vi "Control - PID Control.vi"() -> ()   [LabVIEW 2019, in "Control Workspace Object.lvlib"]
doc: "Sample numeric display item."
uses:
  Control Workspace Object.lvlib
  <vilib>/NI VeriStand/Display Template Support/DisplayTemplateSupport.llb/cluster_Screen Item Settings.ctl
  <vilib>/NI VeriStand/Display Template Support/DisplayTemplateSupport.llb/cluster_Graph Scale Settings.ctl
  <vilib>/NI VeriStand/Display Template Support/DisplayTemplateSupport.llb/cluster_Graph Plot Settings.ctl
  NationalInstruments.VeriStand.SystemStorage
  Shared/Types/Workspace Object State Variables.ctl
  Shared/Types/UI.Refs.ctl
  Shared/Types/UDP Streaming Command Cluster.ctl
  Shared/Types/UDP Streaming State.ctl
  <vilib>/NI VeriStand/Display Template Support/DisplayTemplateSupport.llb/enum_Display Template Handler Minimal To Workspace.ctl
  Shared/Types/Workspace Object Cached Settings.ctl
  <vilib>/NI VeriStand/Execution/Workspace/WorkspaceAPI.ctl
  <vilib>/NI VeriStand/Display Template Support/DisplayTemplateSupport.llb/enum_Display Template Handler Minimal To Widget Msg.ctl
  <vilib>/NI VeriStand/Execution/Workspace/SystemStateRegEventRef.ctl
  <vilib>/NI VeriStand/Execution/Workspace/Target State Info.ctl
  <vilib>/NI VeriStand/Execution/Workspace/Target State.ctl
  <vilib>/NI VeriStand/Execution/Workspace/SystemStateEventRef.ctl
  Shared/Constants.vi
  <vilib>/NI VeriStand/Execution/Workspace/NI VeriStand - Get Multiple Channel Values.vi
  <vilib>/NI VeriStand/Execution/Workspace/NI VeriStand - Set Single Channel Value.vi
  <vilib>/NI VeriStand/Display Template Support/DisplayTemplateSupport.llb/sub_Display Template Handler Custom.vi
  Shared/Control Addon Shared.lvlib
  <vilib>/NI VeriStand/Execution/Workspace/NI_VS Workspace ExecutionAPI.lvlib
  NationalInstruments.VeriStand.ClientAPI
panel:
  in  "Manual Value":bool
  in  "Revert":bool
  in  "Apply":bool
  in  "Manual Output":dbl
  in  "Manual Control":bool
  in  "Setpoint":dbl
  in  "NIVS.System Definition Root":refnum<k24>
  in  "NIVS.Gateway IP Address":string
  in  "Hold":bool
  in  "Autoscale Y":bool=TRUE
  in  "Autoscale X":bool=TRUE
  out "Chart":waveform(dbl)[](graph)
  out "Control Name":string
  in  "Item.Data":T1
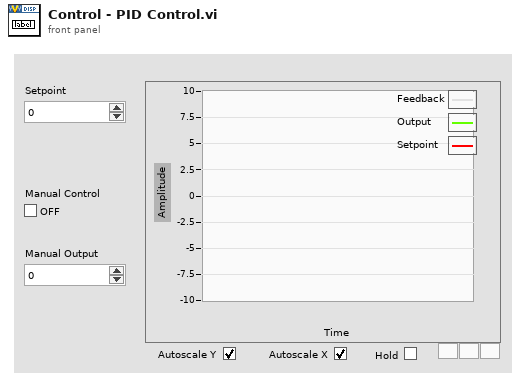
[diagram p1: front panel]
types:
  T1 = typedef "cluster_Screen Item Settings.ctl" = cluster{"Template VI":string, "Position X":i32, "Position Y":i32, "Custom":string, "Show Title Bar":bool, "ID":i32, "Always On Top":bool, "Allow Resize":bool, "Allow Minimize":bool, "Allow Close":bool, "Size to Screen":bool, "Screen.ID":i32, "State":enum16{"Normal", "New"}, "Title":string, "Window Bounds":cluster{"[0]":i16, "[1]":i16, "[2]":i16, "[3]":i16}, "Channel Ref":u64, "Unit":string, "Default Units?":bool, "Flash Limit?":bool, "Color 1":u32, "Color 2":u32, "Color 3":u32, "Color 4":u32, "Bck Color":u32, "Fore Color":u32, "Limit 1":dbl, "Limit 2":dbl, "Limit 3":dbl, "Limit 4":dbl, "Limit Mode 1":i32, "Limit Mode 2":i32, "Limit Mode 3":i32, "Limit Mode 4":i32, "Scale Precision":i32, "Scale Min":dbl, "Scale Max":dbl, "Format":i32, "Precision":i32, "Background Type":i32, "IDs":i32[], "Units":string[], "Labels":string[], "Scale Factor":dbl, "Scale Offset":dbl, "YScale Index":u32[], "XScale":T2, "YScales":T2[], "Plots":T3[], "Update Period":dbl, "History Length":dbl, "My.Ref":refnum<vi>, "Is Control?":bool, "Channel Paths":string[], "Custom Data":variant}
  T2 = typedef "cluster_Graph Scale Settings.ctl" = cluster{"Format":u8, "Precision":u8, "Fit":u8, "Label":string, "Use Default Label":bool, "Label Visible":bool, "Min":dbl, "Max":dbl}
  T3 = typedef "cluster_Graph Plot Settings.ctl" = cluster{"Bar Style":u8, "Fill To":i16, "Fill/PtColor":u32, "Line Style":u8, "Line Width":u8, "Color":u32, "Interp":u8, "Point Style":u8}
  T4 = typedef "Control Addon Shared.lvlib/Workspace Object State Variables.ctl" = cluster{"UI.Refs":T5, "Addon.GUID":string, "Addon.Name":string, "Addon.Type":enum16{"PID", "Industrial"}, "Data.UDPEngineQueue":refnum<queue>, "Data.Found?":bool, "Data.UDPChannels":string[], "Data.PreviousValues":dbl[], "Data.SlowChannels":string[], "Data.PendingChange?":bool, "CachedData.UserEvent":refnum<user-event>, "CachedData.Data":T6, "Workspace.Connected?":bool, "NIVS.SysDef":refnum<k24>, "NIVS.WorkspaceManager":T7, "NIVS.UserEventRefs":cluster{"Event Registration Refnum":refnum<event-registration>, "SystemChangeEventRef":T8}, "NIVS.SystemStateRefs":T9, "NIVS.LaunchRef":refnum<user-event>, "Setpoint Range":cluster{"Min":dbl, "Max":dbl}, "Output Range":cluster{"Min":dbl, "Max":dbl}}
  T5 = typedef "Control Addon Shared.lvlib/UI.Refs.ctl" = cluster{"Chart":refnum<vi>, "Manual Value":refnum<vi>, "Manual Output":refnum<vi>, "Revert":refnum<vi>, "Apply":refnum<vi>, "Setpoint":refnum<vi>, "Autoscale X":refnum<vi>, "Autoscale Y":refnum<vi>, "Hold":refnum<vi>, "Manual Control":refnum<vi>}
  T6 = typedef "Control Addon Shared.lvlib/Workspace Object Cached Settings.ctl" = cluster{"Path":string}
  T7 = typedef "NI_VS Workspace ExecutionAPI.lvlib/WorkspaceAPI.ctl" = refnum<k24>
  T8 = typedef "NI_VS Workspace ExecutionAPI.lvlib/SystemStateRegEventRef.ctl" = refnum<event-registration>
  T9 = typedef "NI_VS Workspace ExecutionAPI.lvlib/SystemStateEventRef.ctl" = cluster{"CustDatRef":refnum<user-event>, "EvtRef":refnum<k27>, "Target State User Event":refnum<user-event>}
  T10 = typedef "enum_Display Template Handler Minimal To Workspace.ctl" = cluster{"Operation":enum16{"SetCustomData", "DeleteItem"}, "Data":variant}
  T11 = typedef "enum_Display Template Handler Minimal To Widget Msg.ctl" = enum16{"Stop", "LaunchConfigDialog"}
  T12 = typedef "Control Addon Shared.lvlib/UDP Streaming Command Cluster.ctl" = cluster{"Action":T13, "Channels":string[]}
  T13 = typedef "Control Addon Shared.lvlib/UDP Streaming State.ctl" = enum8{"Idle", "Start Acq", "Run", "Stop Acq", "Exit"}
  T14 = cluster{"Event Registration Refnum":refnum<event-registration>, "SystemChangeEventRef":T8}
  T15 = typedef "NI_VS Workspace ExecutionAPI.lvlib/SystemState.ctl" = u8
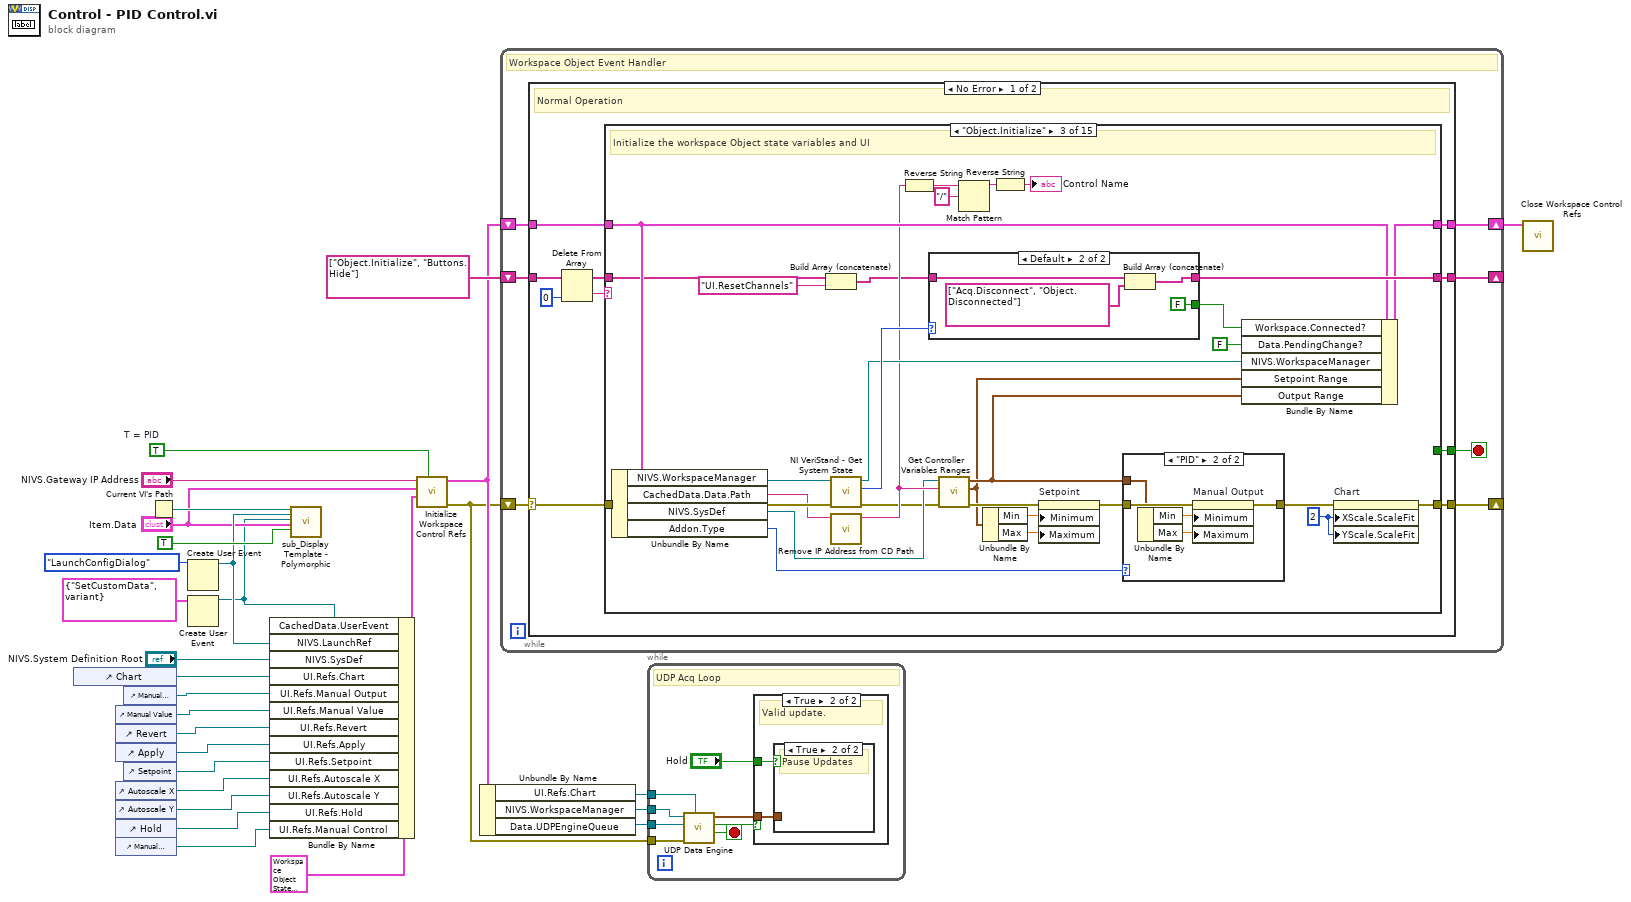
[diagram p0: block diagram]
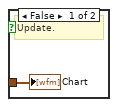
[diagram p3: hidden frame]
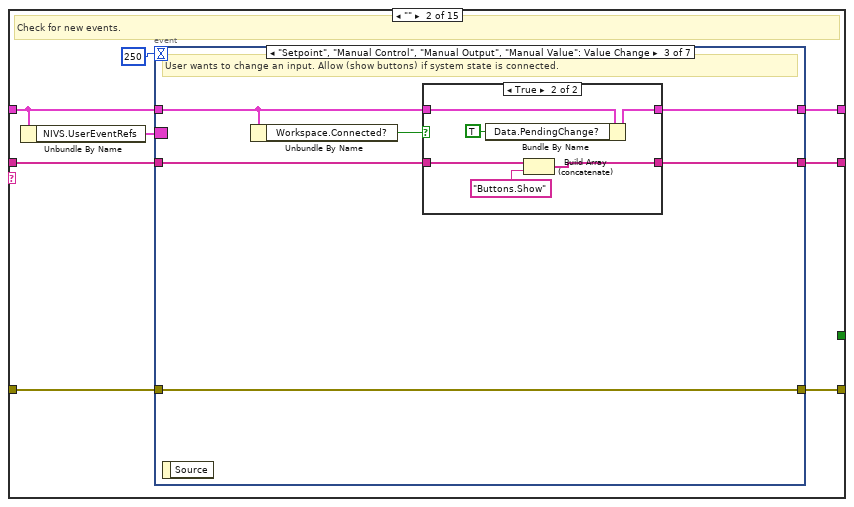
[diagram p5: hidden frame]
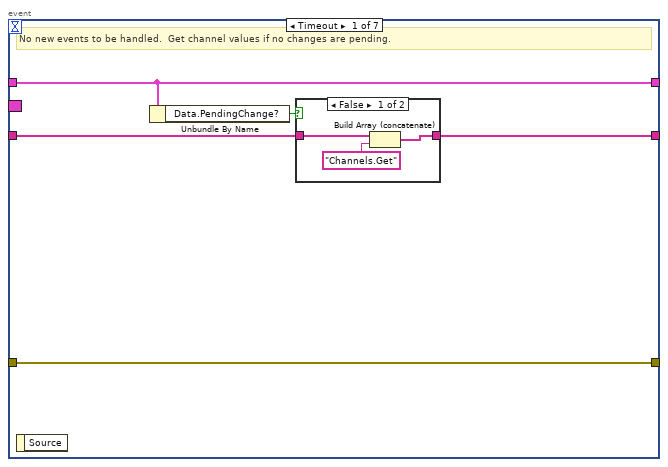
[diagram p6: hidden frame]
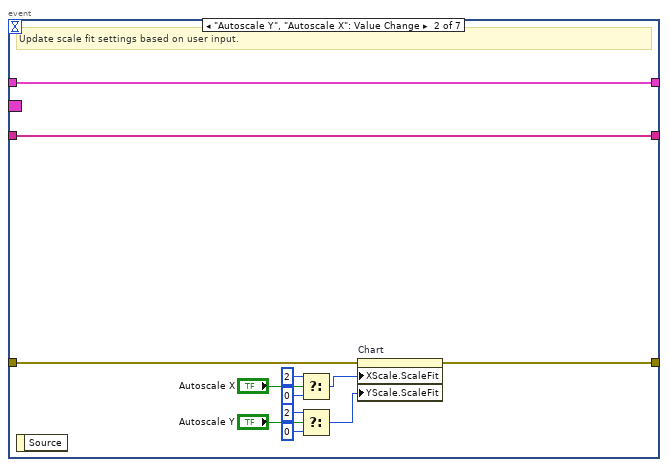
[diagram p8: hidden frame]
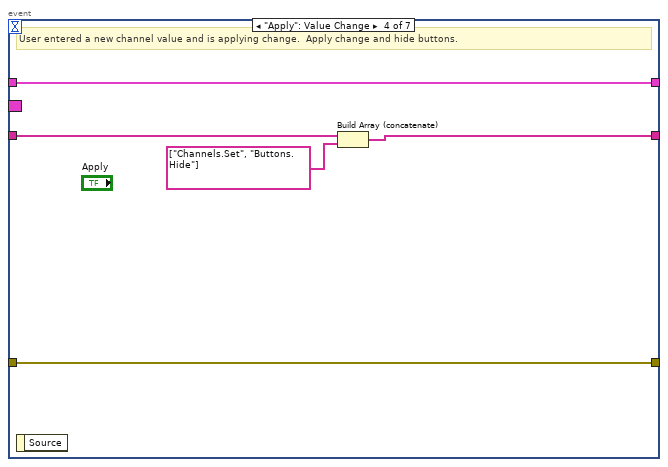
[diagram p10: hidden frame]
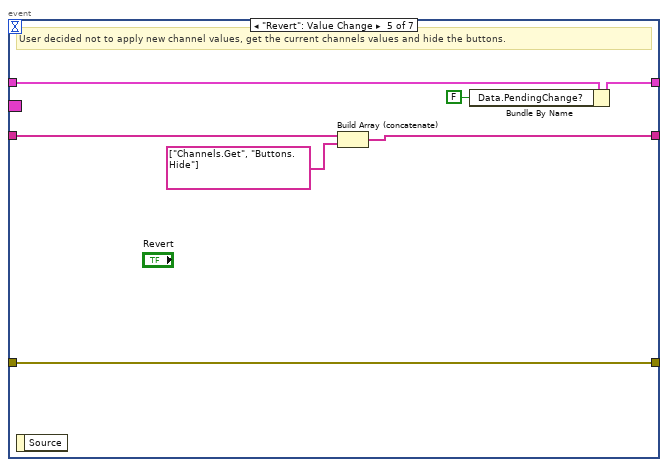
[diagram p11: hidden frame]
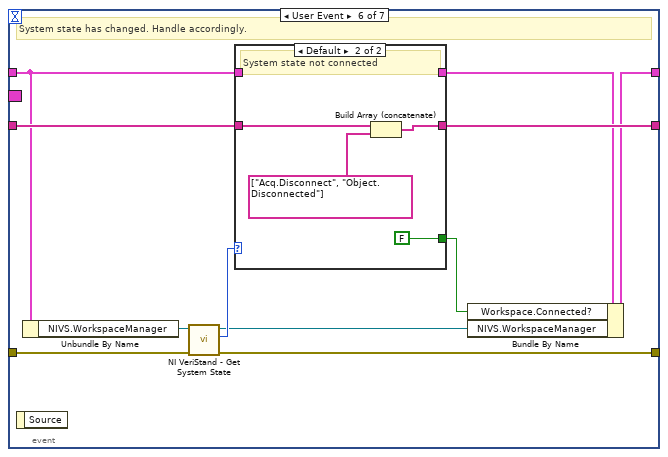
[diagram p12: hidden frame]
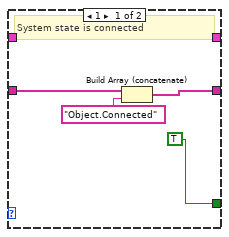
[diagram p13: hidden frame]
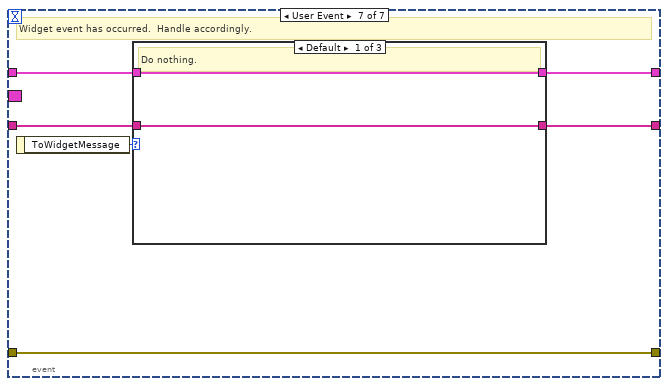
[diagram p14: hidden frame]
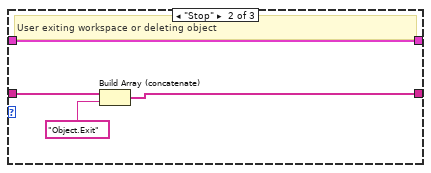
[diagram p15: hidden frame]
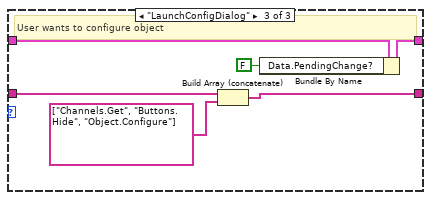
[diagram p16: hidden frame]
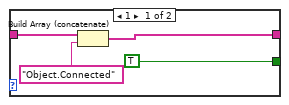
[diagram p18: hidden frame]
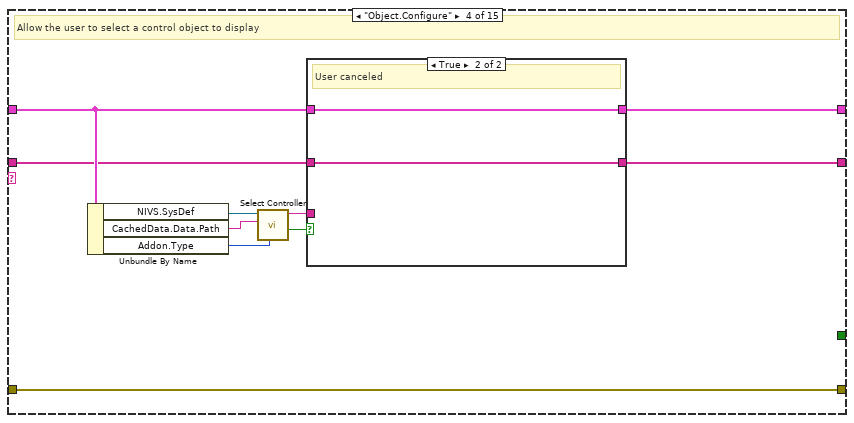
[diagram p19: hidden frame]
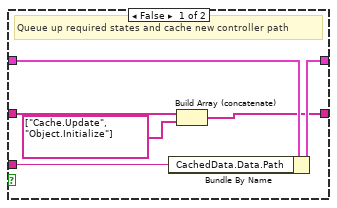
[diagram p20: hidden frame]
diagram:
  w11 = TRUE  # T = PID
  n1 = control-ref of="Chart"() -> (w17:refnum<vi>)
  n2 = control-ref of="Manual Value"() -> (w15:refnum<vi>)
  n3 = control-ref of="Revert"() -> (w14:refnum<vi>)
  n4 = control-ref of="Apply"() -> (w13:refnum<vi>)
  n5 = control-ref of="Autoscale X"() -> (w2:refnum<vi>)
  n6 = control-ref of="Autoscale Y"() -> (w3:refnum<vi>)
  n7 = control-ref of="Hold"() -> (w4:refnum<vi>)
  n8 = control-ref of="Manual Control"() -> (w1:refnum<vi>)
  n9 = control-ref of="Manual Output"() -> (w16:refnum<vi>)
  n10 = control-ref of="Setpoint"() -> (w5:refnum<vi>)
  n11 = Current VI's Path() -> (path=w27:path)
  n12 = Create User Event(user event datatype=enum_Display_Template_Handler_Minimal_To_Widget_Msg."LaunchConfigDialog" ("ToWidgetMessage")) -> (user event=w12:refnum<user-event>)  [unwired: 1 in, 1 out]
  n13 = Create User Event(user event datatype=T10 {"Operation"=enum."SetCustomData", "Data"=variant} ("Data")) -> (user event=w7:refnum<user-event>)  [unwired: 1 in, 1 out]
  n14 = Bundle By Name(cluster=T4 {"UI.Refs"={"Chart"=refnum, "Manual Value"=refnum, "Manual Output"=refnum, "Revert"=refnum, "Apply"=refnum, "Setpoint"=refnum, "Autoscale X"=refnum, "Autoscale Y"=refnum, "Hold"=refnum, "Manual Control"=refnum}, "Addon.GUID"="", "Addon.Name"="", "Addon.Type"=enum."PID", "Data.UDPEngineQueue"=refnum, "Data.Found?"=FALSE, "Data.UDPChannels"=[], "Data.PreviousValues"=[], "Data.SlowChannels"=[], "Data.PendingChange?"=FALSE, "CachedData.UserEvent"=refnum, "CachedData.Data"={"Path"=""}, "Workspace.Connected?"=FALSE, "NIVS.SysDef"=refnum, "NIVS.WorkspaceManager"=refnum, "NIVS.UserEventRefs"={"Event Registration Refnum"=refnum, "SystemChangeEventRef"=refnum}, "NIVS.SystemStateRefs"={"CustDatRef"=refnum, "EvtRef"=refnum, "Target State User Event"=refnum}, "NIVS.LaunchRef"=refnum, "Setpoint Range"={"Min"=0.0, "Max"=0.0}, "Output Range"={"Min"=0.0, "Max"=0.0}}, "CachedData.UserEvent"=w7, "NIVS.LaunchRef"=w12, "NIVS.SysDef"="NIVS.System Definition Root", "UI.Refs.Chart"=w17, "UI.Refs.Manual Output"=w16, "UI.Refs.Manual Value"=w15, "UI.Refs.Revert"=w14, "UI.Refs.Apply"=w13, "UI.Refs.Setpoint"=w5, "UI.Refs.Autoscale X"=w2, "UI.Refs.Autoscale Y"=w3, "UI.Refs.Hold"=w4, "UI.Refs.Manual Control"=w1) -> (w9:T4)
  n15 = call-poly <vilib>:"sub_Display Template - Polymorphic.vi"("Parent.Path"=w27, "ToWidgetEvent"=w12, "ToWorkspace"=w7, "Item.Data"="Item.Data", "Resizable"=TRUE) -> ()  [unwired: 1 in, 14 out]
  n16 = call "Initialize Workspace Control Refs.vi"("T = PID"=w11, "State Variables in"=w9, "Item.Data"="Item.Data", "NIVS.Gateway IP Address"="NIVS.Gateway IP Address") -> ("error out"=w6:errorcluster, "State Variables out"=w20:T4)  [unwired: 6 in]
  n17 = Unbundle By Name(w20) -> ("UI.Refs.Chart"=w22:refnum<vi>, "NIVS.WorkspaceManager"=w21:T7, "Data.UDPEngineQueue"=w19:refnum<queue>)
  n18 = while {
    shift-right: [w34] -> _
    shift-left: string[] ["Object.Initialize", "Buttons.Hide"] -> [w35]
    shift-right: [w32] -> w24
    shift-left: w20 -> [w31]
    shift-right: [w33] -> _
    shift-left: w6 -> [w30]
    stop <- w36 stop-if-true
    # "Workspace Object Event Handler"
    n19 = case shown="No Error" w30 {
      selector: w30 -> [w37 w406]
      tunnel: [w46 _] -> w36
      tunnel: w35 -> [w44 w414]
      tunnel: [w41 w414] -> w34
      tunnel: [w40 w411] -> w33
      tunnel: [w39 w413] -> w32
      tunnel: w31 -> [w38 w413]
      frame No Error {
        # "Normal Operation"
        n20 = Delete From Array(array=w44, index=0) -> (deleted portion=w43:string, array with subset deleted=w42:string[])  [unwired: 1 in]
        n21 = case shown="\"Object.Initialize\"" w43 {
          tunnel: [_ _ _ _ _ _ TRUE _ _ _ _ _ _ _ _] -> w46
          tunnel: [w49 w56 w171 w191 w219 w245 w255 w262 w270 w272 w284 w290 w305 w365 w404] -> w41
          tunnel: w37 -> [w48 w54 w172 w197 w212 w240 w250 w261 w265 w277 w280 w286 w302 w353 w403]
          tunnel: w42 -> [w49 w55 w145 w190 w228 w245 w255 w262 w270 w278 w284 w290 w305 w365 w404]
          tunnel: w38 -> [w47 w50 w162 w195 w227 w242 w247 w258 w269 w274 w283 w289 w295 w351 w402]
          tunnel: [w48 w53 w157 w197 w207 w241 w249 w261 w264 w276 w279 w285 w301 w352 w403] -> w40
          tunnel: [w47 w52 w166 w194 w209 w243 w247 w258 w269 w274 w283 w289 w300 w350 w402] -> w39
          frame Default {
            # "Do nothing."
          }
          frame "" {
            # "Check for new events."
            n22 = Unbundle By Name(w50) -> ("NIVS.UserEventRefs"=w51:T14)
            n23 = event shown="[2] \"Setpoint\", \"Manual Control\", \"Manual Output\", \"Manual Value\": Value Change" {
              selector: w51 -> [_ _ _ _ _ _ _]
              dyn-events: _ -> [_ _ _ _ _ _ _]
              timeout: 250 -> [_ _ _ _ _ _ _]
              tunnel: [w60 w78 w81 w93 w101 w111 w130] -> w56
              tunnel: w55 -> [w61 w78 w82 w94 w102 w112 w129]
              tunnel: w54 -> [w62 w72 w84 w97 w104 w115 w128]
              tunnel: [w62 w71 w84 w97 w104 w114 w128] -> w53
              tunnel: [w59 w77 w83 w96 w99 w110 w126] -> w52
              tunnel: w50 -> [w59 w77 w80 w96 w100 w107 w127]
              event Timeout {
                # "No new events to be handled.  Get channel values if no changes are pending."
                n24 = event-data() -> ()  [unwired: 2 out]
                n25 = Unbundle By Name(w59) -> ("Data.PendingChange?"=w58:bool)
                n26 = case shown="False" w58 {
                  tunnel: w61 -> [w64 w66]
                  tunnel: [w63 w66] -> w60
                  frame False {
                    n27 = Build Array (concatenate)(w64, "Channels.Get") -> (w63:string[])
                  }
                  frame True {
                  }
                }
              }
              event "Autoscale Y", "Autoscale X": Value Change {
                # "Update scale fit settings based on user input."
                n28 = event-data() -> ()  [unwired: 2 out]
                n29 = Select(t=u8 2, s="Autoscale X", f=u8 0 ("X Scale.Scale Fit")) -> (s? t:f=w74:u8)
                n30 = Select(t=u8 2, s="Autoscale Y", f=u8 0 ("X Scale.Scale Fit")) -> (s? t:f=w67:u8)
                n31 = property on="Chart" class="WFChart (strict)"(error in=w72, "XScale.ScaleFit"=w74, "YScale.ScaleFit"=w67) -> (error out=w71:errorcluster)  [unwired: 1 in, 1 out]
              }
              event "Setpoint", "Manual Control", "Manual Output", "Manual Value": Value Change {
                # "User wants to change an input. Allow (show buttons) if system state is connected."
                n32 = event-data() -> ()  [unwired: 2 out]
                n33 = Unbundle By Name(w80) -> ("Workspace.Connected?"=w79:bool)
                n34 = case shown="True" w79 {
                  tunnel: w80 -> [w85 w91]
                  tunnel: [w85 w90] -> w83
                  tunnel: w82 -> [w86 w89]
                  tunnel: [w86 w87] -> w81
                  frame False {
                  }
                  frame True {
                    n35 = Bundle By Name(cluster=w91, "Data.PendingChange?"=TRUE ("Pending Change?")) -> (w90:T4)
                    n36 = Build Array (concatenate)(w89, "Buttons.Show") -> (w87:string[])
                  }
                }
              }
              event "Apply": Value Change {
                # "User entered a new channel value and is applying change.  Apply change and hide buttons."
                n37 = event-data() -> ()  [unwired: 2 out]
                n38 = Build Array (concatenate)(w94, string[] ["Channels.Set", "Buttons.Hide"]) -> (w93:string[])
              }
              event "Revert": Value Change {
                # "User decided not to apply new channel values, get the current channels values and hide the buttons."
                n39 = event-data() -> ()  [unwired: 2 out]
                n40 = Build Array (concatenate)(w102, string[] ["Channels.Get", "Buttons.Hide"]) -> (w101:string[])
                n41 = Bundle By Name(cluster=w100, "Data.PendingChange?"=FALSE ("Pending Change?")) -> (w99:T4)
              }
              event User Event {
                # "System state has changed. Handle accordingly."
                n42 = event-data() -> ()  [unwired: 2 out]
                n43 = Unbundle By Name(w107) -> ("NIVS.WorkspaceManager"=w106:T7)
                n44 = call <vilib>:"NI VeriStand - Get System State.vi"("error in (no error)"=w115, "WorkspaceManager in"=w106) -> ("error out"=w114:errorcluster, "System State"=w113:T15, "WorkspaceManager  out"=w105:T7)  [unwired: 5 in, 2 out]
                n45 = case shown="Default" w113 {
                  tunnel: w112 -> [w120 w125]
                  tunnel: [w119 w124] -> w111
                  tunnel: [w117 w123] -> w109
                  tunnel: w107 -> [w117 w123]
                  tunnel: [TRUE FALSE] -> w108
                  frame 1 {
                    # "System state is connected"
                    n46 = Build Array (concatenate)(w120, "Object.Connected") -> (w119:string[])
                  }
                  frame Default {
                    # "System state not connected"
                    n47 = Build Array (concatenate)(w125, string[] ["Acq.Disconnect", "Object.Disconnected"]) -> (w124:string[])
                  }
                }
                n48 = Bundle By Name(cluster=w109, "Workspace.Connected?"=w108, "NIVS.WorkspaceManager"=w105) -> (w110:T4)
              }
              event User Event {
                # "Widget event has occurred.  Handle accordingly."
                n49 = event-data() -> ("ToWidgetMessage"=w131:T11)  [unwired: 1 out]
                n50 = case shown="Default" w131 {
                  tunnel: [w133 w136 w142] -> w130
                  tunnel: w129 -> [w133 w137 w143]
                  tunnel: w127 -> [w132 w134 w139]
                  tunnel: [w132 w134 w138] -> w126
                  frame Default {
                    # "Do nothing."
                  }
                  frame "Stop" {
                    # "User exiting workspace or deleting object"
                    n51 = Build Array (concatenate)(w137, "Object.Exit") -> (w136:string[])
                  }
                  frame "LaunchConfigDialog" {
                    # "User wants to configure object"
                    n52 = Build Array (concatenate)(w143, string[] ["Channels.Get", "Buttons.Hide", "Object.Configure"]) -> (w142:string[])
                    n53 = Bundle By Name(cluster=w139, "Data.PendingChange?"=FALSE ("Pending Change?")) -> (w138:T4)
                  }
                }
              }
            }
          }
          frame "Object.Initialize" {
            w164 = u8 2 ("X Scale.Scale Fit")
            # "Initialize the workspace Object state variables and UI"
            n54 = Unbundle By Name(w162) -> ("NIVS.WorkspaceManager"=w161:T7, "CachedData.Data.Path"=w155:string, "NIVS.SysDef"=w158:refnum<k24>, "Addon.Type"=w149:enum16{"PID", "Industrial"})
            n55 = Build Array (concatenate)(w145, "UI.ResetChannels") -> (w144:string[])
            n56 = call <vilib>:"NI VeriStand - Get System State.vi"("error in (no error)"=w172, "WorkspaceManager in"=w161) -> ("error out"=w156:errorcluster, "System State"=w173:T15, "WorkspaceManager  out"=w160:T7)  [unwired: 5 in, 2 out]
            n57 = call "Remove IP Address from CD Path.vi"("CD Path"=w155) -> ("Path"=w159:string)  [unwired: 10 in]
            n58 = Reverse String(1:w159) -> (0:w170:string)
            n59 = case shown="Default" w173 {
              tunnel: w144 -> [w183 w187]
              tunnel: [w182 w186] -> w171
              tunnel: [TRUE FALSE] -> w165
              frame 1 {
                n60 = Build Array (concatenate)(w183, "Object.Connected") -> (w182:string[])
              }
              frame Default {
                n61 = Build Array (concatenate)(w187, string[] ["Acq.Disconnect", "Object.Disconnected"]) -> (w186:string[])
              }
            }
            n62 = call "Get Controller Variables Ranges.vi"("error in (no error)"=w156, "Path"=w159, "NIVS.SysDef Ref"=w158) -> ("error out"=w154:errorcluster, "Setpoint Range"=w147:cluster{"Min":dbl, "Max":dbl}, "Output Range"=w148:cluster{"Min":dbl, "Max":dbl})  [unwired: 6 in]
            n63 = Match Pattern(string=w170, regular expression="/") -> (before substring=w167:string)  [unwired: 1 in, 3 out]
            n64 = Unbundle By Name(w147) -> ("Min"=w153:dbl, "Max"=w152:dbl)
            n65 = Reverse String(1:w167) -> (0:→"Control Name":string)
            n66 = property on="Setpoint" class="DigNum (strict)"(error in=w154, "Minimum"=w153, "Maximum"=w152) -> (error out=w151:errorcluster)  [unwired: 1 in, 1 out]
            n67 = case shown="\"PID\"" w149 {
              tunnel: w151 -> [w174 w179]
              tunnel: [w174 w178] -> w150
              tunnel: w148 -> [_ w177]
              frame Default {
              }
              frame "PID" {
                n68 = Unbundle By Name(w177) -> ("Min"=w176:dbl, "Max"=w175:dbl)
                n69 = property on="Manual Output" class="DigNum (strict)"(error in=w179, "Minimum"=w176, "Maximum"=w175) -> (error out=w178:errorcluster)  [unwired: 1 in, 1 out]
              }
            }
            n70 = Bundle By Name(cluster=w162, "Workspace.Connected?"=w165, "Data.PendingChange?"=FALSE ("Pending Change?"), "NIVS.WorkspaceManager"=w160, "Setpoint Range"=w147, "Output Range"=w148) -> (w166:T4)
            n71 = property on="Chart" class="WFChart (strict)"(error in=w150, "XScale.ScaleFit"=w164, "YScale.ScaleFit"=w164) -> (error out=w157:errorcluster)  [unwired: 1 in, 1 out]
          }
          frame "Object.Configure" {
            # "Allow the user to select a control object to display"
            n72 = Unbundle By Name(w195) -> ("NIVS.SysDef"=w189:refnum<k24>, "CachedData.Data.Path"=w196:string, "Addon.Type"=w188:enum16{"PID", "Industrial"})
            n73 = call "Select Controller.vi"("Type"=w188, "CD Path"=w196, "NIVS.System Definition Root"=w189) -> ("Cancelled?"=w193:bool, "Custom Device Path Out"=w192:string)  [unwired: 6 in, 1 out]
            n74 = case shown="True" w193 {
              tunnel: w195 -> [w203 w204]
              tunnel: [w202 w204] -> w194
              tunnel: w192 -> [w201 _]
              tunnel: [w199 w205] -> w191
              tunnel: w190 -> [w200 w205]
              frame False {
                # "Queue up required states and cache new controller path"
                n75 = Bundle By Name(cluster=w203, "CachedData.Data.Path"=w201) -> (w202:T4)
                n76 = Build Array (concatenate)(w200, string[] ["Cache.Update", "Object.Initialize"]) -> (w199:string[])
              }
              frame True {
                # "User canceled"
              }
            }
          }
          frame "Object.Connected" {
            w216 = "/" ("string")
            # "System state is Connected. Get path to required channels and start UDP acquisition if channels found."
            n77 = Unbundle By Name(w227) -> ("NIVS.SysDef"=w213:refnum<k24>, "CachedData.Data.Path"=w226:string, "Addon.Name"=w214:string, "Addon.GUID"=w211:string)
            n78 = global read "Constants.vi" "Name.ManualControl"() -> (w225:string)
            n79 = global read "Constants.vi" "Name.Channels"() -> (w215:string)
            n80 = call "Remove IP Address from CD Path.vi"("CD Path"=w226) -> ("Path"=w224:string)  [unwired: 10 in]
            n81 = Concatenate Strings(w224, w216, w215, w216, w225) -> (w223:string)
            n82 = Concatenate Strings(w224, w216, w215, w216, w214) -> (w222:string)
            n83 = call "Get Dependent Nodes from SysDef Root.vi"("error in (no error)"=w212, "GUID"=w211, "Path"=w224, "SysDef Ref"=w213) -> ("error out"=w208:errorcluster, "Channels"=w218:string[], "Found"=w206:bool)  [unwired: 5 in]
            n84 = Index Array(array=w218, index=2) -> (element=w220:string)
            n85 = Build Array(w220, w223, w222) -> (w217:string[])
            n86 = Bundle By Name(cluster=w227, "Data.Found?"=w206, "Data.UDPChannels"=w218, "Data.SlowChannels"=w217) -> (w210:T4)
            n87 = case shown="True" w206 {
              tunnel: w228 -> [w229 w239]
              tunnel: [w229 w238] -> w219
              tunnel: w210 -> [w230 w237]
              tunnel: [w230 w236] -> w209
              tunnel: w208 -> [w231 w235]
              tunnel: [w231 w234] -> w207
              frame False {
              }
              frame True {
                n88 = call "UI Set DisableState.vi"("Enable?"=TRUE, "error in (no error)"=w235, "State Variables in"=w237) -> ("error out"=w234:errorcluster, "State Variables out"=w236:T4)  [unwired: 7 in]
                n89 = Build Array (concatenate)(w239, "Acq.Start") -> (w238:string[])
              }
            }
          }
          frame "Object.Disconnected" {
            n90 = call "UI Set DisableState.vi"("Enable?"=FALSE, "error in (no error)"=w240, "State Variables in"=w242) -> ("error out"=w241:errorcluster, "State Variables out"=w243:T4)  [unwired: 7 in]
          }
          frame "Object.Exit" {
            # "Stop current loop.  Queue Stop Acq and Exit to UDP loop."
            n91 = Unbundle By Name(w247) -> ("Data.UDPEngineQueue"=w246:refnum<queue>)
            n92 = Enqueue Element(queue=w246, element=T12 {"Action"=enum."Stop Acq", "Channels"=[]}, error in (no error)=w250) -> (queue out=w253:refnum<queue>, error out=w251:errorcluster)  [unwired: 1 in, 1 out]
            n93 = Enqueue Element(queue=w253, element=T12 {"Action"=enum."Exit", "Channels"=[]}, error in (no error)=w251) -> (error out=w249:errorcluster)  [unwired: 1 in, 2 out]
          }
          frame "Cache.Update" {
            # "Cache any data needing to be permenantly stored with the workspace object."
            n94 = Unbundle By Name(w258) -> ("CachedData.UserEvent"=w256:refnum<user-event>, "CachedData.Data"=w257:T6)
            n95 = Bundle By Name(cluster=T10 {"Operation"=enum."SetCustomData", "Data"=variant} ("event data"), "Data"=w257) -> (w259:T10)
            n96 = Generate User Event(user event=w256, event data cluster=w259) -> ()  [unwired: 2 in, 2 out]
          }
          frame "Acq.Start" {
            # "Send a Start Acq command to the UDP Loop.  Include the channels to  monitor."
            n97 = Unbundle By Name(w269) -> ("Data.UDPEngineQueue"=w263:refnum<queue>, "Data.UDPChannels"=w267:string[])
            n98 = Bundle By Name(cluster=T12 {"Action"=enum."Start Acq", "Channels"=[]}, "Channels"=w267) -> (w266:T12)
            n99 = Enqueue Element(queue=w263, element=w266, error in (no error)=w265) -> (error out=w264:errorcluster)  [unwired: 1 in, 2 out]
          }
          frame "Acq.Disconnect" {
            # "Send Stop Acq to the UDP Acq Loop.  Reset the UI."
            n100 = Unbundle By Name(w274) -> ("Data.UDPEngineQueue"=w273:refnum<queue>)
            n101 = Enqueue Element(queue=w273, element=T12 {"Action"=enum."Stop Acq", "Channels"=[]}, error in (no error)=w277) -> (error out=w276:errorcluster)  [unwired: 1 in, 2 out]
            n102 = Build Array (concatenate)(w278, "UI.ResetChannels") -> (w272:string[])
          }
          frame "Buttons.Hide" {
            w281 = FALSE ("Hold")
            # "Hide the apply and revert buttons from the user."
            n103 = property on="Apply" class="Bool"(error in=w280, "Visible"=w281) -> (error out=w282:errorcluster)  [unwired: 1 in, 1 out]
            n104 = property on="Revert" class="Bool"(error in=w282, "Visible"=w281) -> (error out=w279:errorcluster)  [unwired: 1 in, 1 out]
          }
          frame "Buttons.Show" {
            w287 = TRUE ("Hold")
            # "Show the apply and revert buttons to the user."
            n105 = property on="Apply" class="Bool"(error in=w286, "Visible"=w287) -> (error out=w288:errorcluster)  [unwired: 1 in, 1 out]
            n106 = property on="Revert" class="Bool"(error in=w288, "Visible"=w287) -> (error out=w285:errorcluster)  [unwired: 1 in, 1 out]
          }
          frame "Channels.Get" {
            # "Get the current slow speed channel values from VeriStand if no pending change, data paths are valid and system state is connected."
            n107 = Unbundle By Name(w295) -> ("Setpoint Range.Max"=w294:dbl, "Setpoint Range.Min"=w293:dbl, "Data.PendingChange?"=w296:bool, "Output Range.Max"=w292:dbl, "Output Range.Min"=w291:dbl, "Addon.Type"=w299:enum16{"PID", "Industrial"}, "Data.Found?"=w303:bool, "Workspace.Connected?"=w304:bool, "NIVS.WorkspaceManager"=w298:T7, "Data.SlowChannels"=w297:string[])
            n108 = case shown="False" w296 {
              tunnel: w304 -> [w327 _]
              tunnel: w303 -> [w321 _]
              tunnel: w302 -> [w318 w344]
              tunnel: [w317 w344] -> w301
              tunnel: [w316 w345] -> w300
              tunnel: w299 -> [w315 _]
              tunnel: w298 -> [w314 _]
              tunnel: w297 -> [w312 _]
              tunnel: w295 -> [w311 w345]
              tunnel: w294 -> [w309 _]
              tunnel: w293 -> [w308 _]
              tunnel: w292 -> [w307 _]
              tunnel: w291 -> [w306 _]
              frame False {
                # "No pending data change.  Allow for a get."
                n109 = Compound Arithmetic op=AND(w321, w327) -> (w322:bool)
                n110 = case shown="True" w322 {
                  tunnel: w318 -> [w337 w343]
                  tunnel: [w337 w342] -> w317
                  tunnel: w314 -> [w336 w341]
                  tunnel: [w336 w340] -> w313
                  tunnel: w312 -> [_ w339]
                  tunnel: [dbl[] [0.0, 0.0, 0.0] ("Values") w338] -> w326
                  frame False {
                    # "Do Nothing."
                  }
                  frame True {
                    # "Connected & paths valid"
                    n111 = call-poly <vilib>:"NI VeriStand - Get Channel Value.vi"("error in (no error)"=w343, "Channels"=w339, "WorkspaceManager in"=w341) -> ("error out"=w342:errorcluster, "Values"=w338:dbl[], "WorkspaceManager out"=w340:T7)  [unwired: 6 in]
                  }
                }
                n112 = Index Array(array=w326) -> (element #1=w325:dbl, element #2=w320:dbl, element #3=w319:dbl)  [unwired: 3 in]
                n113 = case shown="\"PID\"" w315 {
                  tunnel: w319 -> [w329 w334]
                  tunnel: w307 -> [_ w332]
                  tunnel: w306 -> [_ w331]
                  frame "Industrial" {
                    n114 = To Long Integer(number=w329) -> (32bit integer=w330:i32)
                    n115 = Not Equal To 0?(x=w330) -> (x != 0?=w328:bool)
                    n116 = local write "Manual Value"(w328) -> ()
                  }
                  frame "PID" {
                    n117 = In Range and Coerce(upper limit=w332, x=w334, lower limit=w331) -> (coerced(x)=w333:dbl)  [unwired: 1 out]
                    n118 = local write "Manual Output"(w333) -> ()
                  }
                }
                n119 = To Long Integer(number=w320) -> (32bit integer=w324:i32)
                n120 = In Range and Coerce(upper limit=w309, x=w325, lower limit=w308) -> (coerced(x)=w310:dbl)  [unwired: 1 out]
                n121 = Not Equal To 0?(x=w324) -> (x != 0?=w323:bool)
                n122 = local write "Setpoint"(w310) -> ()
                n123 = local write "Manual Control"(w323) -> ()
                n124 = Bundle By Name(cluster=w311, "NIVS.WorkspaceManager"=w313, "Data.PreviousValues"=w326) -> (w316:T4)
              }
              frame True {
                # "A change is pending.  Don't get channels as this would overwrite the pending change."
              }
            }
          }
          frame "Channels.Set" {
            # "Set Channels if data paths are valid and system state is connected and there is a change in the data value."
            n125 = Unbundle By Name(w351) -> ("Data.Found?"=w356:bool, "Workspace.Connected?"=w359:bool, "Data.PreviousValues"=w358:dbl[], "Data.SlowChannels"=w360:string[], "NIVS.WorkspaceManager"=w348:T7, "Addon.Type"=w346:enum16{"PID", "Industrial"})
            n126 = case shown="\"PID\"" w346 {
              tunnel: [w367 "Manual Output"] -> w354
              frame "Industrial" {
                n127 = Boolean To (0,1)(Boolean="Manual Value") -> (0, 1=w367:i16)
              }
              frame "PID" {
              }
            }
            n128 = Boolean To (0,1)(Boolean="Manual Control") -> (0, 1=w355:i16)
            n129 = Build Array("Setpoint", w355, w354) -> (w361:dbl[])
            n130 = Not Equal?(x=w358, y=w361) -> (x != y?=w364:bool[])
            n131 = Compound Arithmetic op=AND(w356, w359) -> (w357:bool)
            n132 = case shown="True" w357 {
              tunnel: w364 -> [_ w377]
              tunnel: w361 -> [_ w376]
              tunnel: w353 -> [w370 w375]
              tunnel: [w370 w374] -> w352
              tunnel: w348 -> [w369 w373]
              tunnel: [w369 w372] -> w347
              tunnel: w360 -> [_ w371]
              frame False {
                # "Do nothing"
              }
              frame True {
                # "Connected & paths valid"
                n133 = for {
                  shift-right: [w383] -> w374
                  shift-left: w375 -> [w384]
                  shift-right: [w382] -> w372
                  shift-left: w373 -> [w381]
                  tunnel: w377 -> [w380] mode=indexing
                  tunnel: w376 -> [w379] mode=indexing
                  tunnel: w371 -> [w378] mode=indexing
                  n134 = case shown="False" w380 {
                    tunnel: w384 -> [w386 w392]
                    tunnel: [w386 w391] -> w383
                    tunnel: [w385 w390] -> w382
                    tunnel: w381 -> [w385 w389]
                    tunnel: w379 -> [_ w388]
                    tunnel: w378 -> [_ w387]
                    frame False {
                      # "Do nothing"
                    }
                    frame True {
                      # "Update channel"
                      n135 = call-poly <vilib>:"NI VeriStand - Set Channel Value.vi"("error in (no error)"=w392, "Value"=w388, "Channel"=w387, "WorkspaceManager in"=w389) -> ("error out"=w391:errorcluster, "WorkspaceManager out"=w390:T7)  [unwired: 6 in]
                    }
                  }
                }
              }
            }
            n136 = Bundle By Name(cluster=w351, "Data.PendingChange?"=FALSE ("Pending Change?"), "NIVS.WorkspaceManager"=w347) -> (w350:T4)
          }
          frame "UI.ResetChannels" {
            w394 = TRUE ("Manual Control")
            w393 = FALSE ("Manual Control")
            w397 = 0.0 ("Setpoint")
            # "Reset slow speed channel displayed values."
            n137 = Unbundle By Name(w402) -> ("Setpoint Range.Max"=w401:dbl, "Setpoint Range.Min"=w400:dbl, "Output Range.Max"=w399:dbl, "Output Range.Min"=w398:dbl)
            n138 = In Range and Coerce(upper limit=w401, x=w397, lower limit=w400) -> (coerced(x)=w396:dbl)  [unwired: 1 out]
            n139 = In Range and Coerce(upper limit=w399, x=w397, lower limit=w398) -> (coerced(x)=w395:dbl)  [unwired: 1 out]
            n140 = local write "Setpoint"(w396) -> ()
            n141 = local write "Manual Output"(w395) -> ()
            n142 = local write "Manual Control"(w393) -> ()
            n143 = local write "Manual Value"(w393) -> ()
            n144 = local write "Hold"(w393) -> ()
            n145 = local write "Autoscale X"(w394) -> ()
            n146 = local write "Autoscale Y"(w394) -> ()
          }
        }
      }
      frame Error {
        # "Handle Errors."
        n147 = Unbundle By Name(w406) -> ("code"=w410:i32)
        n148 = Equal?(x=-307654, y=w410) -> (x = y?=w408:bool)
        n149 = Select(t=errorcluster {"status"=FALSE, "code"=0, "source"=""}, s=w408, f=w406) -> (s? t:f=w405:errorcluster)
        n150 = call <vilib>:"Simple Error Handler.vi"("error in (no error)"=w405) -> ("error out"=w412:errorcluster)  [unwired: 4 in, 4 out]
        n151 = call <vilib>:"Clear Errors.vi"("error in (no error)"=w412) -> ("error out"=w411:errorcluster)  [unwired: 5 in, 1 out]
      }
    }
  }
  n152 = while {
    tunnel: w21 -> [w417]
    tunnel: w19 -> [w422]
    tunnel: w22 -> [w418]
    tunnel: w6 -> [w416]
    stop <- w421 stop-if-true
    # "UDP Acq Loop"
    n153 = call "UDP Data Engine.vi"("WaveformChart Ref"=w418, "error in (no error)"=w416, "UDP Engine Queue"=w422, "WorkspaceManager"=w417) -> ("Exit"=w421:bool, "Update?"=w415:bool, "Waveform"=w419:waveform(dbl)[])  [unwired: 4 in, 1 out]
    n154 = case shown="True" w415 {
      tunnel: "Hold" -> [_ w424]
      tunnel: w419 -> [_ w423]
      frame False {
        # "Do Nothing."
      }
      frame True {
        # "Valid update."
        n155 = case shown="True" w424 {
          tunnel: w423 -> [w425 _]
          frame False {
            # "Update."
            "Chart" <- w425
          }
          frame True {
            # "Pause Updates"
          }
        }
      }
    }
  }
  n156 = call "Close Workspace Control Refs.vi"("State Variables in"=w24) -> ()  [unwired: 11 in]
